vi "dispose.vi"(8 "error in":errorcluster, 11 "websocket client in":refnum<class "websocket client.lvclass">) -> (0 "error out":errorcluster)   [LabVIEW 2016, in "websocket client.lvclass"]
uses:
  websocket client.lvclass
  websocket client.lvclass/websocket client.ctl
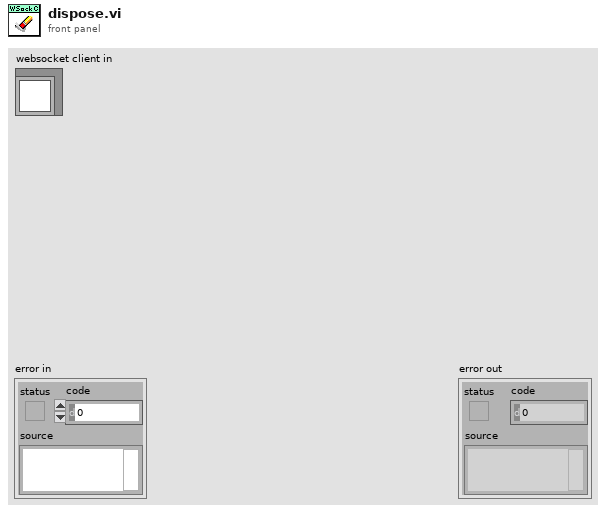
[diagram p1: front panel]
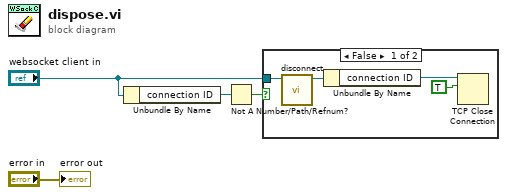
[diagram p0: block diagram]
diagram:
  n1 = Unbundle By Name("websocket client in") -> ("connection ID"=w4:refnum<k5>)
  n2 = Not A Number/Path/Refnum?(number/path/refnum=w4) -> (NaN/Path/Refnum?=w3:bool)
  n3 = case shown="False" w3 {
    tunnel: "websocket client in" -> [w8 _]
    frame False {
      n4 = call "disconnect.vi"("websocket client in"=w8) -> ("websocket client out"=w7:refnum<class "websocket client.lvclass">)  [unwired: 8 in, 2 out]
      n5 = Unbundle By Name(w7) -> ("connection ID"=w6:refnum<k5>)
      n6 = TCP Close Connection(connection ID=w6, abort (F)=TRUE) -> ()  [unwired: 1 in, 2 out]
    }
    frame True {
    }
  }
  "error out" <- "error in"
